vi "Part 2.vi"(11 "Input":string) -> (3 "Output":i64)   [LabVIEW 2021]
uses:
  <userlib>/_OpenG.lib/string/string.llb/Convert EOLs (String)__ogtk.vi
panel:
  in  "Multiplier":i64=1000000
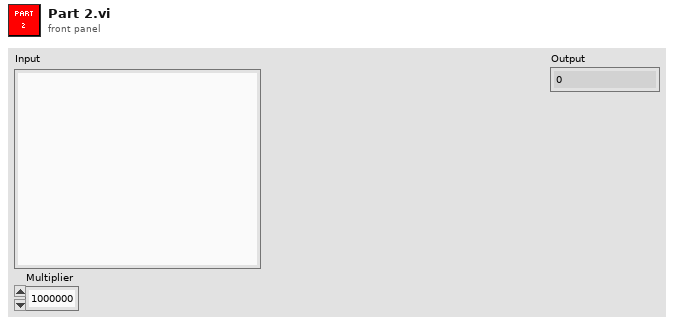
[diagram p1: front panel]
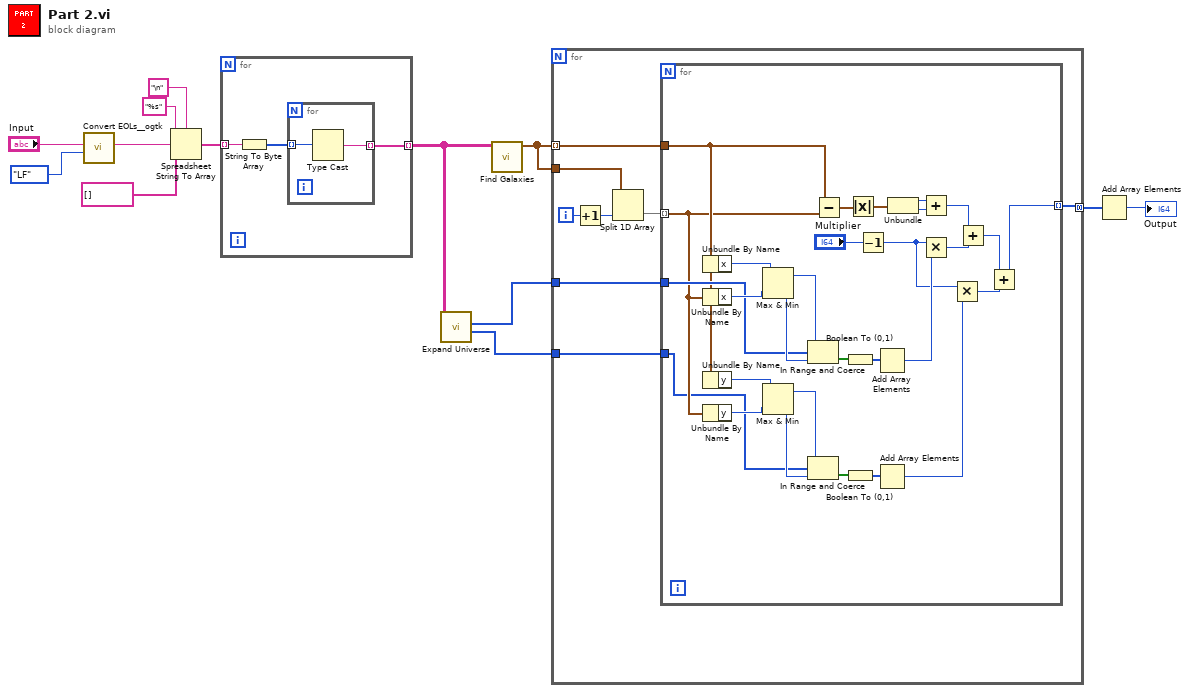
[diagram p0: block diagram]
diagram:
  n1 = call-poly <userlib>:"Convert EOLs__ogtk.vi"("Convert to:"=enum16{"CR", "LF", "CRLF"}."LF", "String in"="Input") -> ("String out"=w9:string)  [unwired: 9 in]
  n2 = Spreadsheet String To Array(delimiter (Tab)="\n", format string="%s", spreadsheet string=w9, array type (2D Dbl)=string[] []) -> (array=w7:string[])
  n3 = for {
    tunnel: w7 -> [w16] mode=indexing
    tunnel: [w14] -> w3 mode=indexing
    n4 = String To Byte Array(string=w16) -> (unsigned byte array=w15:u8[])
    n5 = for {
      tunnel: w15 -> [w18] mode=indexing
      tunnel: [w17] -> w14 mode=indexing
      n6 = Type Cast(x=w18) -> (*(type *) &x=w17:string)  [unwired: 1 in]
    }
  }
  n7 = call "Expand Universe.vi"("Univers In"=w3) -> ("Expandable Columns"=w1:i32[], "Expandable Rows"=w2:i32[])  [unwired: 8 in, 1 out]
  n8 = call "Find Galaxies.vi"("Universe In"=w3) -> ("Galaxies"=w6:cluster{"x":i32, "y":i32}[])  [unwired: 10 in]
  n9 = for {
    tunnel: w6 -> [w22] mode=indexing
    tunnel: w6 -> [w26]
    tunnel: [w21] -> w5 mode=concatenating
    tunnel: w2 -> [w20]
    tunnel: w1 -> [w19]
    i -> [w25]
    n10 = Increment(x=w25) -> (x+1=w24:i32)
    n11 = Split 1D Array(array=w26, index=w24) -> (second subarray=w23:cluster{"x":i32, "y":i32}[])  [unwired: 1 out]
    n12 = for {
      tunnel: w23 -> [w31] mode=indexing
      tunnel: w22 -> [w32]
      tunnel: [w47] -> w21 mode=indexing
      tunnel: w20 -> [w41]
      tunnel: w19 -> [w30]
      n13 = Unbundle By Name(w32) -> ("x"=w45:i32)
      n14 = Unbundle By Name(w31) -> ("x"=w44:i32)
      n15 = Unbundle By Name(w32) -> ("y"=w28:i32)
      n16 = Unbundle By Name(w31) -> ("y"=w33:i32)
      n17 = Max & Min(x=w45, y=w44) -> (max(x,y)=w43:i32, min(x,y)=w42:i32)
      n18 = Max & Min(x=w28, y=w33) -> (max(x,y)=w34:i32, min(x,y)=w35:i32)
      n19 = In Range and Coerce(upper limit=w43, x=w41, lower limit=w42) -> (In Range?=w40:bool[])  [unwired: 1 out]
      n20 = In Range and Coerce(upper limit=w34, x=w30, lower limit=w35) -> (In Range?=w36:bool[])  [unwired: 1 out]
      n21 = Subtract(x=w32, y=w31) -> (x-y=w55:cluster{"x":i32, "y":i32})
      n22 = Boolean To (0,1)(Boolean=w40) -> (0, 1=w39:i16[])
      n23 = Boolean To (0,1)(Boolean=w36) -> (0, 1=w37:i16[])
      n24 = Absolute Value(x=w55) -> (abs(x)=w54:cluster{"x":i32, "y":i32})
      n25 = Decrement(x="Multiplier") -> (x-1=w27:i64)
      n26 = Add Array Elements(numeric array=w39) -> (sum=w38:i16)
      n27 = Add Array Elements(numeric array=w37) -> (sum=w29:i16)
      n28 = Unbundle(w54) -> ("x"=w53:i32, "y"=w52:i32)
      n29 = Add(x=w53, y=w52) -> (x+y=w51:i32)
      n30 = Multiply(x=w27, y=w38) -> (x*y=w50:i64)
      n31 = Multiply(x=w27, y=w29) -> (x*y=w49:i64)
      n32 = Add(x=w51, y=w50) -> (x+y=w48:i64)
      n33 = Add(x=w48, y=w49) -> (x+y=w47:i64)
    }
  }
  n34 = Add Array Elements(numeric array=w5) -> (sum=→"Output":i64)
